vi "Simulation Statechart.vi"(5 "firstStep?":bool, 7 "enableVisualization?":bool=TRUE, 8 "error in":errorcluster, 10 "sensors":T1={"net distance (mm)"=0, "net angle (deg)"=0, "accelerometer"={"x axis (g)"=0.0, "y axis (g)"=0.0, "z axis (g)"=0.0}, "iRobot Sensors"={"Bumps + Wheel Drops"={"Wheeldrop Caster"=FALSE, "Wheeldrop Left"=FALSE, "Wheeldrop Right"=FALSE, "Bump Left"=FALSE, "Bump Right"=FALSE}, "Wall"=FALSE, "Cliff Left"=FALSE, "Cliff Front Left"=FALSE, "Cliff Front Right"=FALSE, "Cliff Right"=FALSE, "Wall Signal"=0, "Cliff Left Signal"=0, "Cliff Front Left Signal"=0, "Cliff Front Right Signal"=0, "Cliff Right Signal"=0, "Buttons"={"Advance"=FALSE, "Play"=FALSE}, "Virtual Wall"=FALSE, "# Stream Packets"=0, "Requested Velocity (mm/s)"=0, "Requested Radius (mm)"=0, "Requested Right Wheel Velocity (mm/s)"=0, "Requested Left Wheel Velocity (mm/s)"=0, "Distance (mm)"=0, "Angle (deg)"=0, "Song Playing"=FALSE, "Song Number"=0, "Charging State"=enum."Not Charging", "Voltage (mV)"=0, "Current (mA)"=0, "Battery Temperature (deg C)"=0, "Battery Charge (mAh)"=0, "Battery Capacity (mAh)"=0, "Charging Sources"={"Internal Charger"=FALSE, "Home Base"=FALSE}, "OI Mode"=enum."Off", "Digital Inputs"={"Digital Input 0"=FALSE, "Digital Input 1"=FALSE, "Digital Input 2"=FALSE, "Digital Input 3"=FALSE, "Device Detect"=FALSE}, "Drivers & Wheel Overcurrent"={"Low-Side Driver 0"=FALSE, "Low-Side Driver 1"=FALSE, "Low-Side Driver 2"=FALSE, "Left Wheel"=FALSE, "Right Wheel"=FALSE}, "Analog Signal"=0, "Infrared"=255}, "Is Simulator?"=FALSE} {"iRobot Sensors"."Infrared" format="%02x"; "accelerometer"."z axis (g)" format="%.3f"; "accelerometer"."y axis (g)" format="%.3f"; "accelerometer"."x axis (g)" format="%.3f"}) -> (0 "error out":errorcluster, 1 "Diagram Display":picture, 2 "sensors":T1={"net distance (mm)"=0, "net angle (deg)"=0, "accelerometer"={"x axis (g)"=0.0, "y axis (g)"=0.0, "z axis (g)"=0.0}, "iRobot Sensors"={"Bumps + Wheel Drops"={"Wheeldrop Caster"=FALSE, "Wheeldrop Left"=FALSE, "Wheeldrop Right"=FALSE, "Bump Left"=FALSE, "Bump Right"=FALSE}, "Wall"=FALSE, "Cliff Left"=FALSE, "Cliff Front Left"=FALSE, "Cliff Front Right"=FALSE, "Cliff Right"=FALSE, "Wall Signal"=0, "Cliff Left Signal"=0, "Cliff Front Left Signal"=0, "Cliff Front Right Signal"=0, "Cliff Right Signal"=0, "Buttons"={"Advance"=FALSE, "Play"=FALSE}, "Virtual Wall"=FALSE, "# Stream Packets"=0, "Requested Velocity (mm/s)"=0, "Requested Radius (mm)"=0, "Requested Right Wheel Velocity (mm/s)"=0, "Requested Left Wheel Velocity (mm/s)"=0, "Distance (mm)"=0, "Angle (deg)"=0, "Song Playing"=FALSE, "Song Number"=0, "Charging State"=enum."Not Charging", "Voltage (mV)"=0, "Current (mA)"=0, "Battery Temperature (deg C)"=0, "Battery Charge (mAh)"=0, "Battery Capacity (mAh)"=0, "Charging Sources"={"Internal Charger"=FALSE, "Home Base"=FALSE}, "OI Mode"=enum."Off", "Digital Inputs"={"Digital Input 0"=FALSE, "Digital Input 1"=FALSE, "Digital Input 2"=FALSE, "Digital Input 3"=FALSE, "Device Detect"=FALSE}, "Drivers & Wheel Overcurrent"={"Low-Side Driver 0"=FALSE, "Low-Side Driver 1"=FALSE, "Low-Side Driver 2"=FALSE, "Left Wheel"=FALSE, "Right Wheel"=FALSE}, "Analog Signal"=0, "Infrared"=255}, "Is Simulator?"=FALSE} {"iRobot Sensors"."Infrared" format="%02x"; "accelerometer"."z axis (g)" format="%.3f"; "accelerometer"."y axis (g)" format="%.3f"; "accelerometer"."x axis (g)" format="%.3f"})   [LabVIEW 2013]
uses:
  shared/Sensors.ctl
  iRobot/Sensor/Accelerometer.ctl
  iRobot/Sensor/Sensor Group 6.ctl
  iRobot/Sensor/Bumps + Wheel Drops.ctl
  iRobot/Sensor/Buttons.ctl
  iRobot/Sensor/Charging State.ctl
  iRobot/Sensor/Charging Sources Available.ctl
  iRobot/Sensor/OI Mode.ctl
  iRobot/Sensor/Cargo Bay Digital Inputs.ctl
  iRobot/Sensor/Low-Side Driver + Wheel Overcurrent.ctl
  Statechart.lvsc/StatechartState.ctl
  Statechart.lvsc/State.ctl
  Statechart.lvsc/CompanionDiagram.vi/42/SC Main.vi
  Statechart.lvsc/CompanionDiagram.vi/42/Upd State.vi
  Statechart.lvsc/CompanionDiagram.vi/42/Trans Graph0.vi
  Statechart.lvsc/CompanionDiagram.vi/42/EnterGraphCore.vi
  Statechart.lvsc/CompanionDiagram.vi/42/Trans Graph1.vi
  Statechart.lvsc/CompanionDiagram.vi/42/Trans Graph2.vi
  Statechart.lvsc/CompanionDiagram.vi
  shared/Wrap Angle.vi
  Statechart.lvsc/Trigger.ctl
  <vilib>/Statechart/Infrastructure/RTStatechart/RunTime SCN.xnode
  Statechart.lvsc/Inputs.ctl
  Statechart.lvsc/Outputs.ctl
  Statechart.lvsc
panel:
  # "Electrical: charging, battery, OI mode"
  # "Sensors: bump, cliff, button, wheel drop, wall, virtual wall"
  # "Motion: distance, angle, requested velocity"
  # "Cargo Bay: I/O, overcurrent, infrared"
  # "Song"
  # "Electrical: charging, battery, OI mode"
  # "Sensors: bump, cliff, button, wheel drop, wall, virtual wall"
  # "Motion: distance, angle, requested velocity"
  # "Cargo Bay: I/O, overcurrent, infrared"
  # "Song"
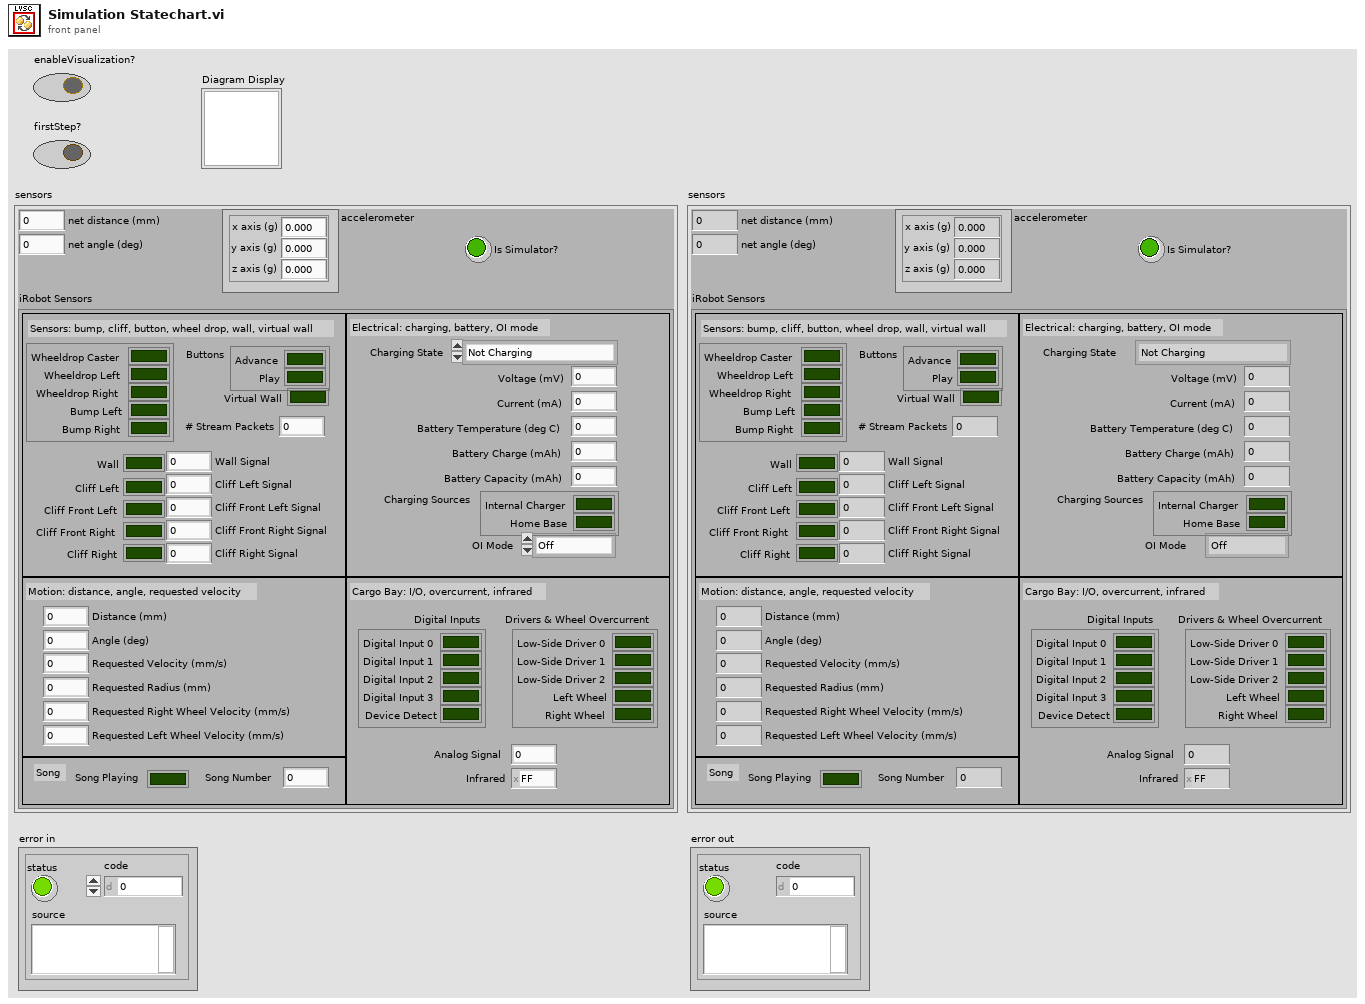
[diagram p1: front panel]
types:
  T1 = typedef "Sensors.ctl" = cluster{"net distance (mm)":i32, "net angle (deg)":i32, "accelerometer":T2, "iRobot Sensors":T3, "Is Simulator?":bool}
  T2 = typedef "Accelerometer.ctl" = cluster{"x axis (g)":dbl, "y axis (g)":dbl, "z axis (g)":dbl}
  T3 = typedef "Sensor Group 6.ctl" = cluster{"Bumps + Wheel Drops":T4, "Wall":bool, "Cliff Left":bool, "Cliff Front Left":bool, "Cliff Front Right":bool, "Cliff Right":bool, "Wall Signal":u16, "Cliff Left Signal":u16, "Cliff Front Left Signal":u16, "Cliff Front Right Signal":u16, "Cliff Right Signal":u16, "Buttons":T5, "Virtual Wall":bool, "# Stream Packets":u8, "Requested Velocity (mm/s)":i16, "Requested Radius (mm)":i16, "Requested Right Wheel Velocity (mm/s)":i16, "Requested Left Wheel Velocity (mm/s)":i16, "Distance (mm)":i32, "Angle (deg)":i32, "Song Playing":bool, "Song Number":u8, "Charging State":T6, "Voltage (mV)":u16, "Current (mA)":i16, "Battery Temperature (deg C)":i8, "Battery Charge (mAh)":u16, "Battery Capacity (mAh)":u16, "Charging Sources":T7, "OI Mode":T8, "Digital Inputs":T9, "Drivers & Wheel Overcurrent":T10, "Analog Signal":u16, "Infrared":u8}
  T4 = typedef "Bumps + Wheel Drops.ctl" = cluster{"Wheeldrop Caster":bool, "Wheeldrop Left":bool, "Wheeldrop Right":bool, "Bump Left":bool, "Bump Right":bool}
  T5 = typedef "Buttons.ctl" = cluster{"Advance":bool, "Play":bool}
  T6 = typedef "Charging State.ctl" = enum16{"Not Charging", "Reconditioning Charging", "Full Charging", "Trickle Charging", "Waiting", "Charging Fault Condition"}
  T7 = typedef "Charging Sources Available.ctl" = cluster{"Internal Charger":bool, "Home Base":bool}
  T8 = typedef "OI Mode.ctl" = enum16{"Off", "Passive", "Safe", "Full"}
  T9 = typedef "Cargo Bay Digital Inputs.ctl" = cluster{"Digital Input 0":bool, "Digital Input 1":bool, "Digital Input 2":bool, "Digital Input 3":bool, "Device Detect":bool}
  T10 = typedef "Low-Side Driver + Wheel Overcurrent.ctl" = cluster{"Low-Side Driver 0":bool, "Low-Side Driver 1":bool, "Low-Side Driver 2":bool, "Left Wheel":bool, "Right Wheel":bool}
  T11 = typedef "Statechart.lvsc/StatechartState.ctl" = T12[]
  T12 = typedef "Statechart.lvsc/State.ctl" = enum16{"NI.SC.Initial", "NI.SC.History", "NI.SC.ShallowHistory", "NI.SC.Terminal", "Pause", "Run", "Pause\\Detect Play Button\\Pause;\nWait for\nbutton\nrelease", "Pause\\Detect Play Button\\Unpause;\nwait for\nbutton release", "Pause\\Detect Play Button\\Unpause;\nwait for\nbutton press", "Run\\Run Mode\\Turn", "Run\\Run Mode\\Drive"}
  T13 = typedef "Statechart.lvsc/Outputs.ctl" = cluster{"Left Wheel Speed (mm/s)":i16, "Right Wheel Speed (mm/s)":i16}
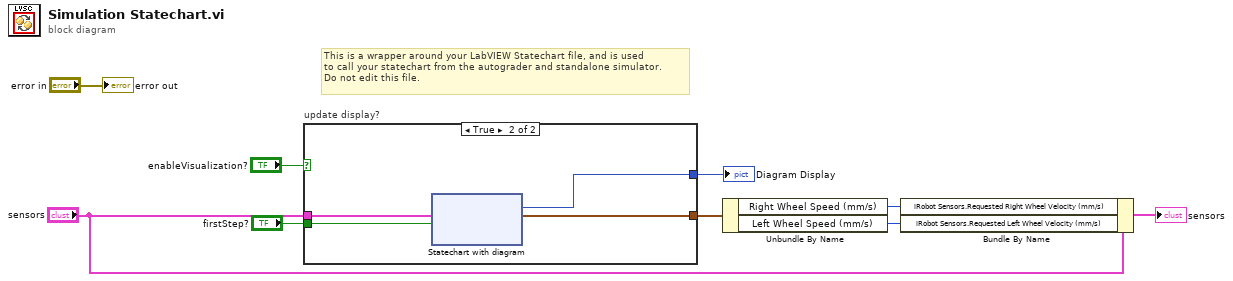
[diagram p0: block diagram]
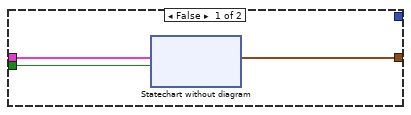
[diagram p2: hidden frame]
diagram:
  # "This is a wrapper around your LabVIEW Statechart file, and is used\nto call your statechart from the autograder and standalone simulator.\nDo not edit this file."
  n1 = case "update display?" shown="True" "enableVisualization?" {
    tunnel: "sensors" -> [w10 w18]
    tunnel: [w11 w21] -> w5
    tunnel: "firstStep?" -> [w12 w20]
    tunnel: [_ w19] -> w4
    frame False {
      n2 = xnode "Statechart without diagram"("Init?"=w12, "Inputs"=w10) -> ("Outputs"=w11:T13)  [unwired: 1 in, 1 out]
    }
    frame True {
      n3 = xnode "Statechart with diagram"("Init?"=w20, "Inputs"=w18) -> ("Outputs"=w21:T13, "Diagram Display"=w19:picture)  [unwired: 2 in, 1 out]
    }
  }
  "Diagram Display" <- w4
  n4 = Unbundle By Name(w5) -> ("Right Wheel Speed (mm/s)"=w7:i16, "Left Wheel Speed (mm/s)"=w6:i16)
  n5 = Bundle By Name(cluster="sensors", "iRobot Sensors.Requested Right Wheel Velocity (mm/s)"=w7, "iRobot Sensors.Requested Left Wheel Velocity (mm/s)"=w6) -> (→"sensors":T1)
  "error out" <- "error in"
